vi "auto_sl.vi"() -> ()   [LabVIEW 2012, in "Mecanum Drive.lvrbt"]
uses:
  Mecanum Drive.lvrbt
  SubVIs/State_Typ.ctl
  <vilib>/NXT/HiTechnic/HiTechnic Controls/HiTechnic Port.ctl
  <vilib>/NXT/Block Support/NXT_InputPort.ctl
  SubVIs/auto_drive_TYP.ctl
  <vilib>/NXT/Hardware/Plugins/Tetrix DC Motor/TetrixDCMotorAddress.ctl
  <vilib>/NXT/Dual Mode Library/Display/drawNumber.vi
  <vilib>/NXT/NXTIO Xnodes/NXTIONodeSubVIs/TETRIX IO Check Battery.vi
  <vilib>/NXT/Dual Mode Library/Waits/Wait_Num(msec).vi
  <vilib>/NXT/NXTIO Xnodes/NXTIONodeSubVIs/TETRIX IO Reset Encoders.vi
  <vilib>/NXT/NXTIO Xnodes/NXTIONodeSubVIs/TETRIX IO Motor Status.vi
  <vilib>/NXT/NXTIO Xnodes/NXTIONodeSubVIs/TETRIX IO Stop DC Motors.vi
  <vilib>/NXT/Dual Mode Library/Sound/Tone.vi
  <vilib>/NXT/Dual Mode Library/Waits/Wait_Num.vi
  <vilib>/NXT/Subs/LVHSConnector.ctl
  <vilib>/NXT/NXTIO Xnodes/AddressXNode/NXTIOAddress.xnode
  <vilib>/NXT/NXTIO Xnodes/NXTIOXNode/NXTIO.xnode
  <vilib>/NXT/LegoClasses/BrickReference/BrickReference.lvclass
panel:
  out "Enabled":bool
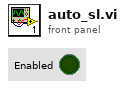
[diagram p1: front panel]
types:
  T1 = typedef "auto_drive_TYP.ctl" = cluster{"Left X":i8, "Left Y":i8, "Right X":i8, "Power (100)":i8, "Wait (ms)":u32, "Enc/Deg Target":i32, "Move Type":enum16{"Relative Degrees", "Wait", "Encoder"}}
  T2 = typedef "State_Typ.ctl" = enum16{"Stop", "Check for Position 3", "Check for Position 2", "Move", "Reset Enc", "Read Enc"}
  T3 = typedef "HiTechnic Port.ctl" = cluster{"Port":T4, "MUX Port":u8}
  T4 = typedef "NXT_InputPort.ctl" = u32
  T5 = typedef "TetrixDCMotorAddress.ctl" = i32
  T6 = typedef "LVHSConnector.ctl" = refnum<class "BrickReference.lvclass">
  T7 = cluster{"TetrixDCMotor":T5, "TetrixDCMotor 2":T5}
  T8 = cluster{"Direction (0-9)":i16, "Signal Strength (Array)":u8[]}
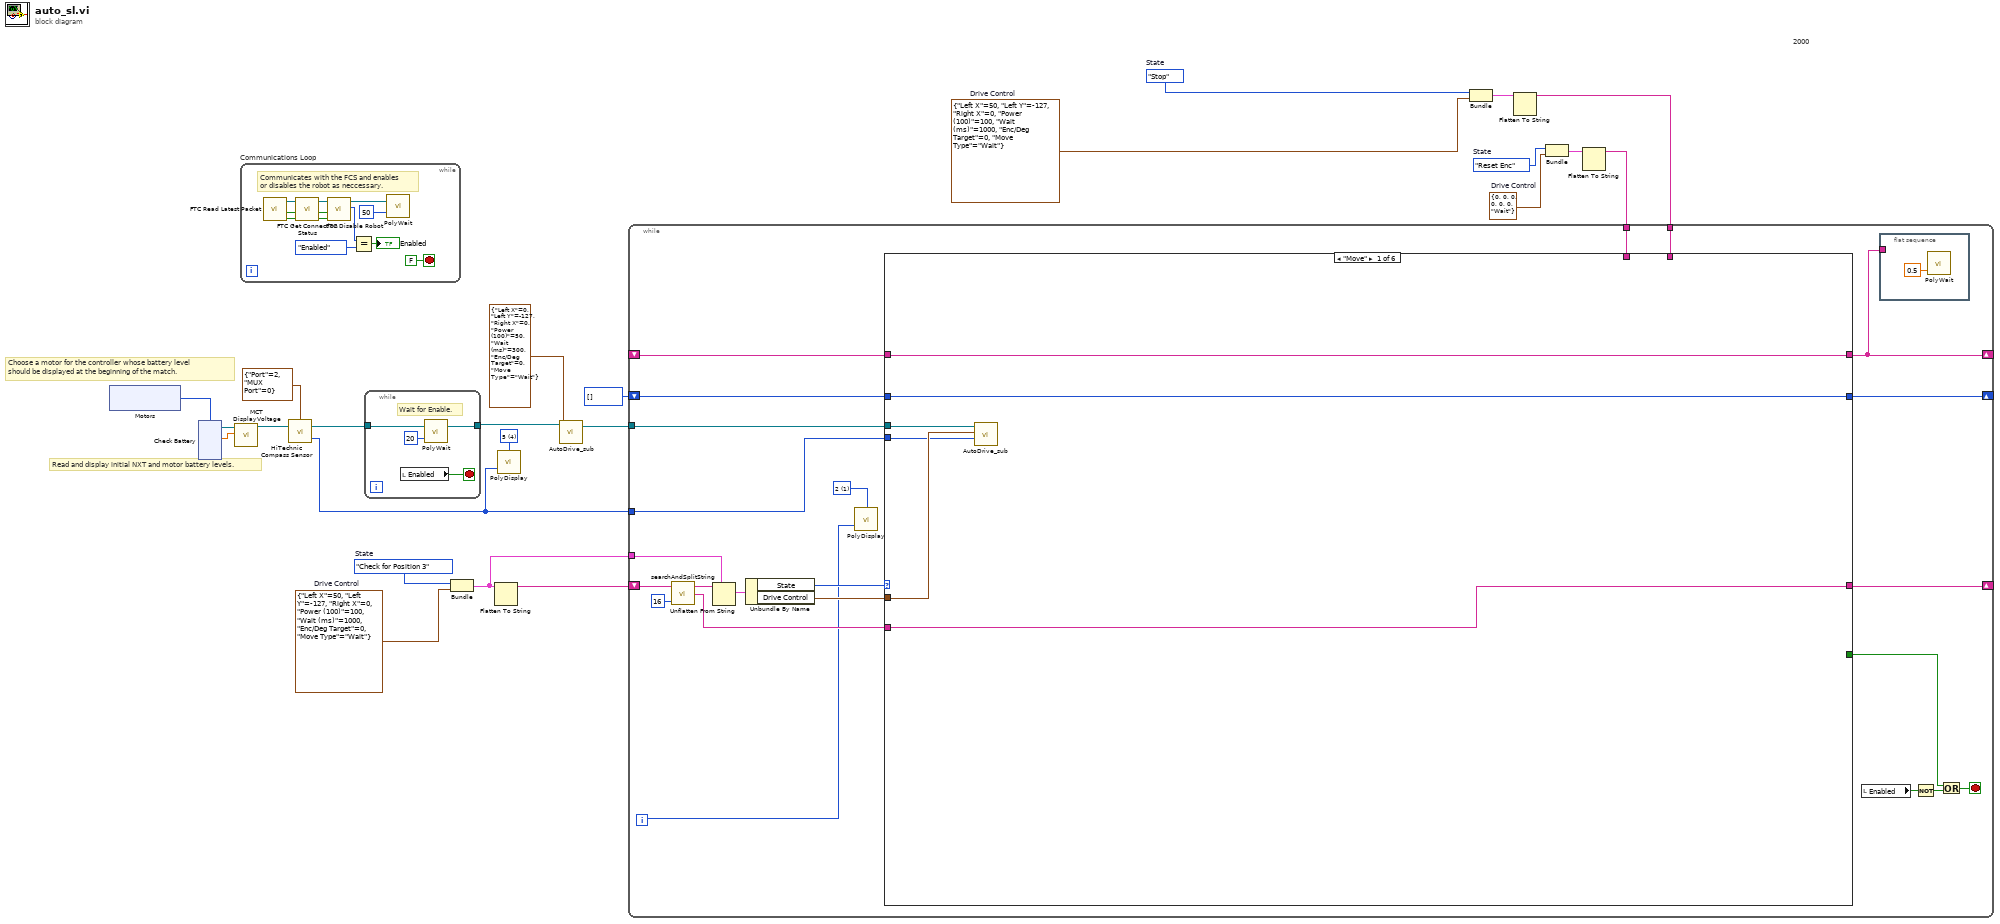
[diagram p0: block diagram]
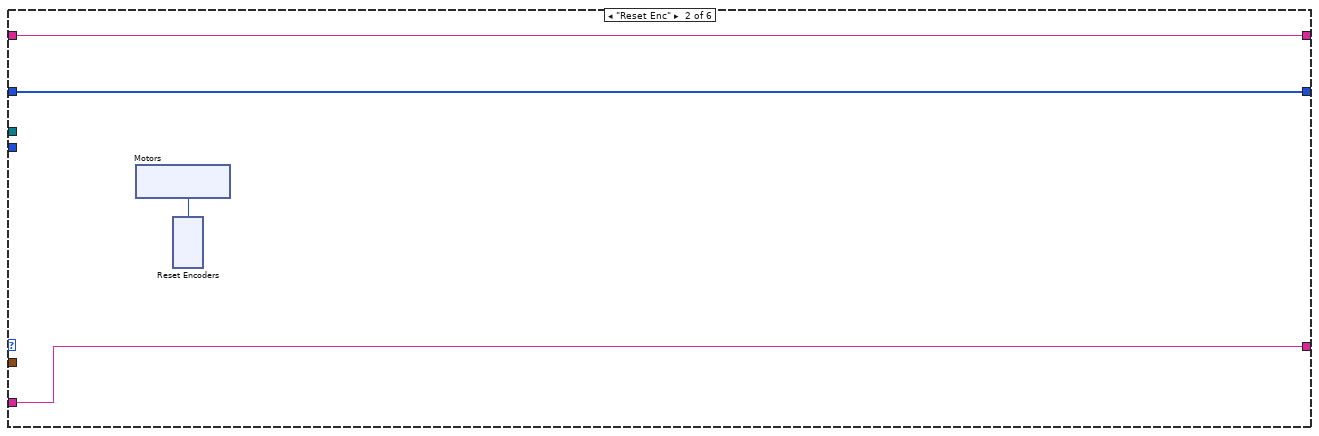
[diagram p2: hidden frame]
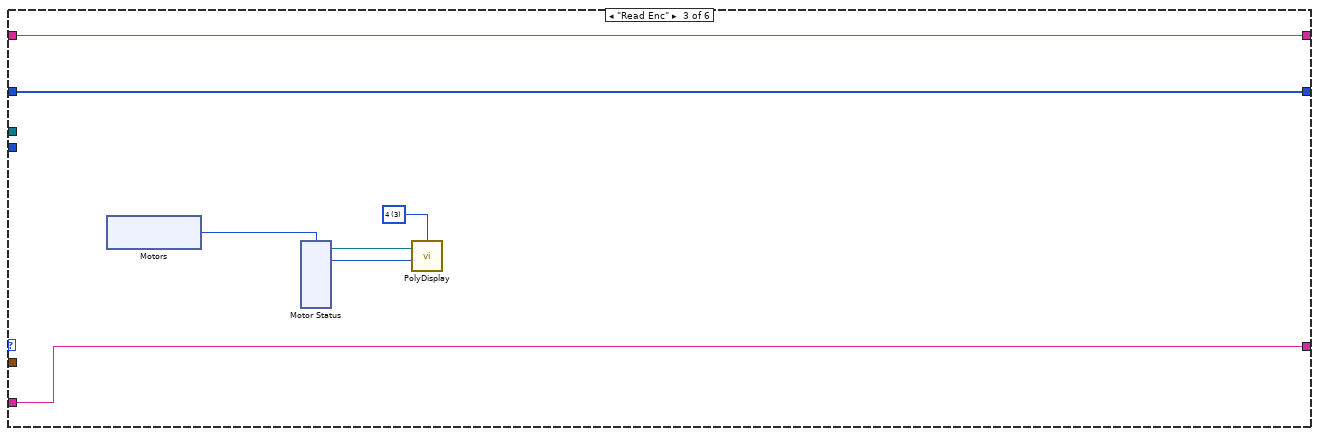
[diagram p3: hidden frame]
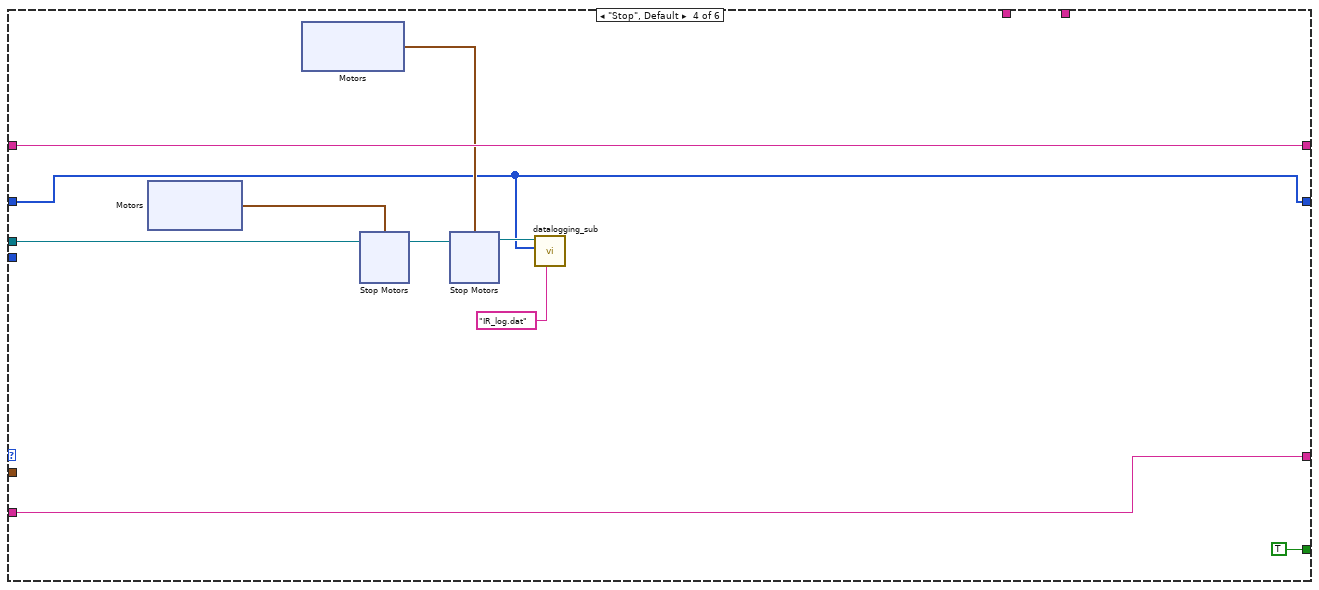
[diagram p4: hidden frame]
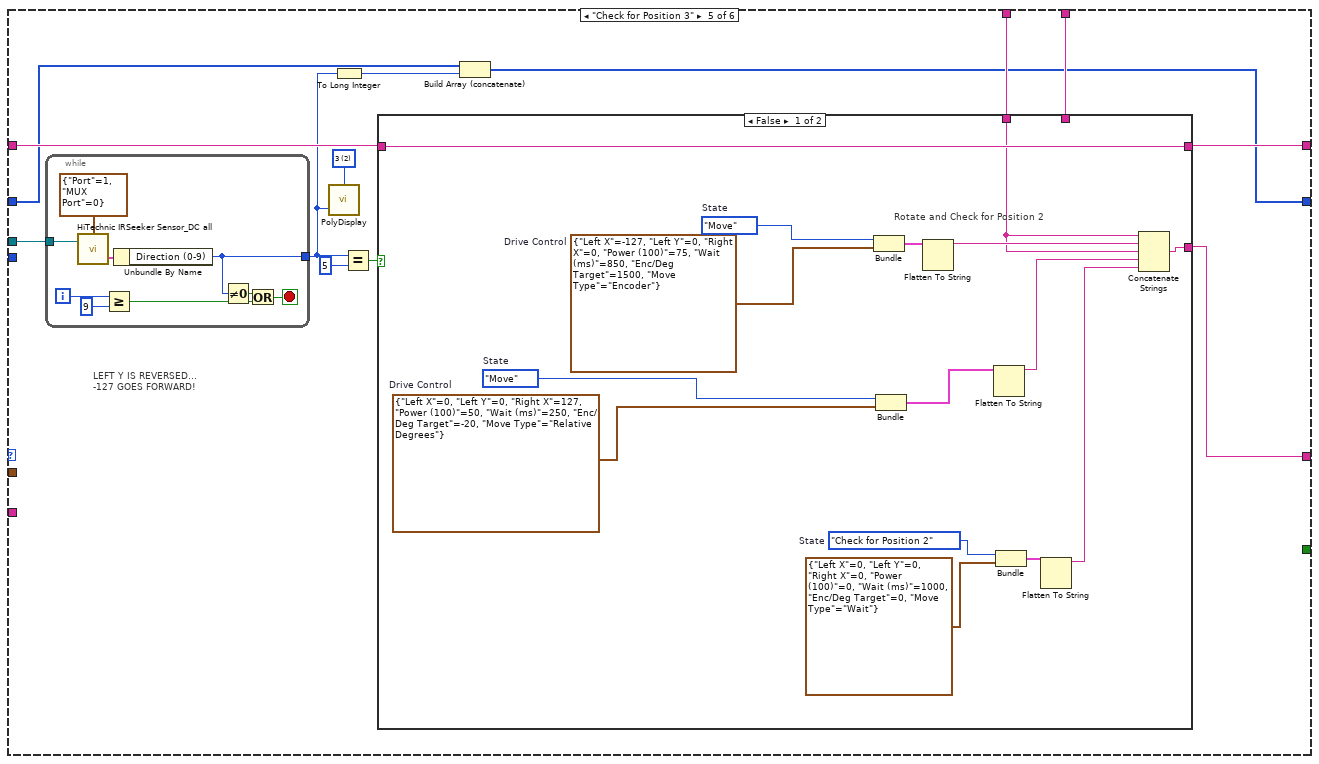
[diagram p5: hidden frame]
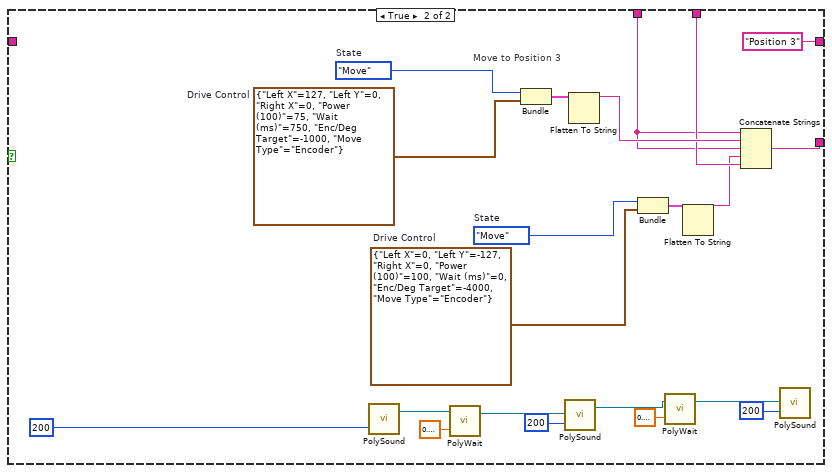
[diagram p6: hidden frame]
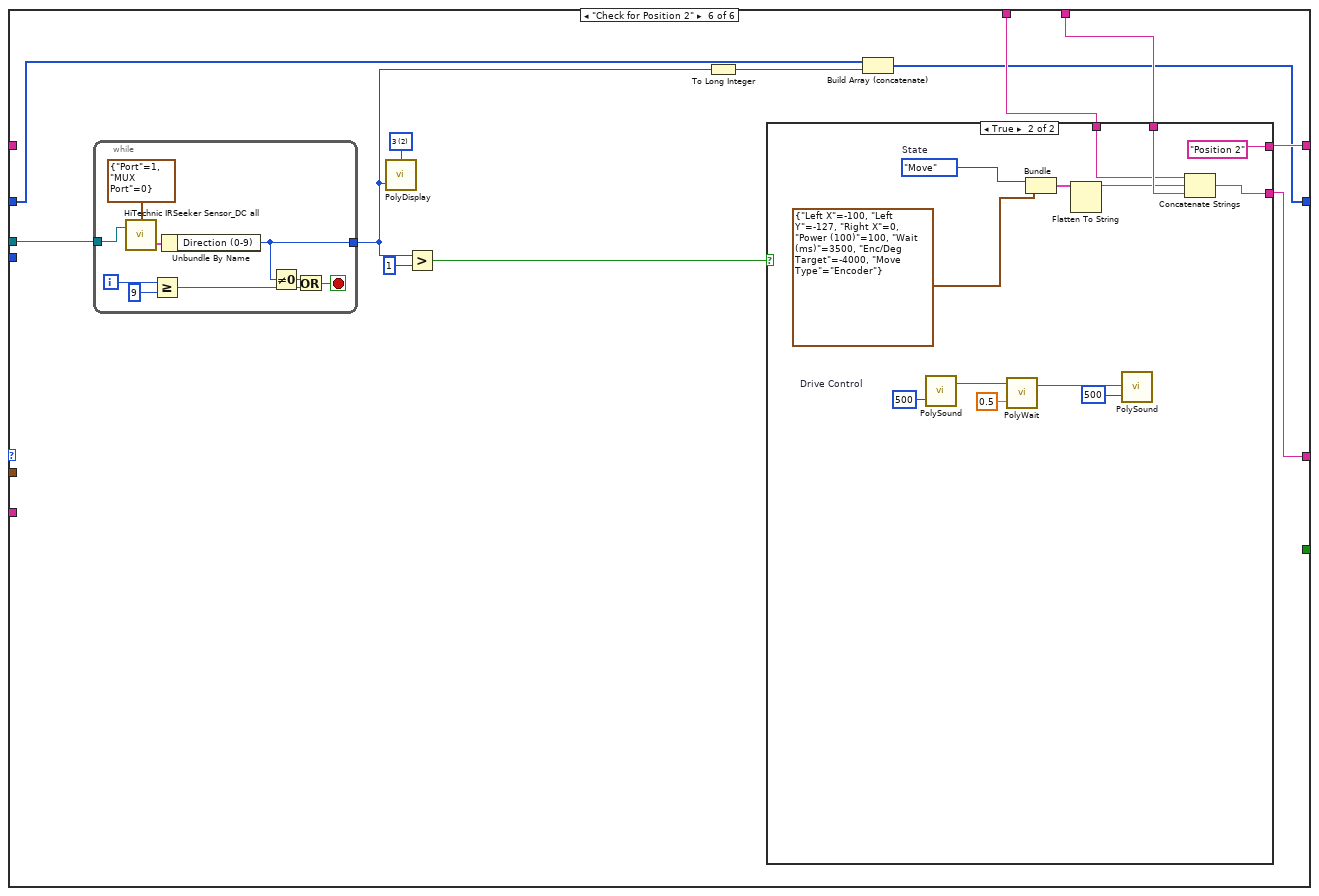
[diagram p7: hidden frame]
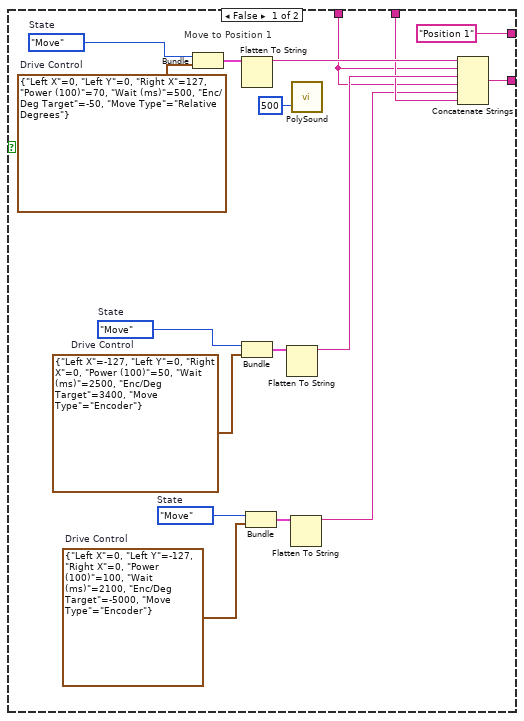
[diagram p8: hidden frame]
diagram:
  w1 = T1 {"Left X"=0, "Left Y"=0, "Right X"=0, "Power (100)"=0, "Wait (ms)"=0, "Enc/Deg Target"=0, "Move Type"=enum."Wait"}  # Drive Control
  w3 = State_Typ."Reset Enc"  # State
  w11 = T1 {"Left X"=50, "Left Y"=-127, "Right X"=0, "Power (100)"=100, "Wait (ms)"=1000, "Enc/Deg Target"=0, "Move Type"=enum."Wait"}  # Drive Control
  w12 = State_Typ."Stop"  # State
  w15 = i16 4 items=["1", "2", "3", "4", "5", "6", "7", "8", "9", "10", "11", "12"] ("Line")
  w24 = T1 {"Left X"=50, "Left Y"=-127, "Right X"=0, "Power (100)"=100, "Wait (ms)"=1000, "Enc/Deg Target"=0, "Move Type"=enum."Wait"}  # Drive Control
  w23 = State_Typ."Check for Position 3"  # State
  # "2000"
  # "Read and display initial NXT and motor battery levels."
  # "Choose a motor for the controller whose battery level \nshould be displayed at the beginning of the match."
  n1 = xnode "Motors"() -> ("Motor"=w20:T5)
  n2 = xnode "Check Battery"("Motors"=w20) -> ("Voltage 1"=w21:sgl, "NXT/EV3"=w22:T6)  [unwired: 1 in]
  n3 = call <vilib>:"MCT DisplayVoltage.vi"("Motor Voltage"=w21, "NXT"=w22) -> ("NXT"=w16:T6)  [unwired: 9 in]
  n4 = while "Communications Loop" {
    stop <- FALSE stop-if-true
    # "Communicates with the FCS and enables \nor disables the robot as neccessary."
    n5 = call <vilib>:"FTC Read Latest Packet.vi"() -> ("Packet Received?"=w34:bool, "Stopped?"=w33:bool, "NXT"=w36:T6)  [unwired: 6 in, 3 out]
    n6 = call <vilib>:"FTC Get Connection Status.vi"("Packet Received?"=w34, "Stopped?"=w33, "NXT"=w36) -> ("Online?"=w25:bool, "Stopped?"=w26:bool, "NXT"=w35:T6)  [unwired: 5 in]
    n7 = call <vilib>:"FTC Disable Robot.vi"("Online?"=w25, "Stopped?"=w26, "NXT"=w35) -> ("Enabled?"=w29:enum16{"Disabled", "Enabled"}, "NXT"=w31:T6)  [unwired: 3 in]
    n8 = Equal?(x=w29, y=enum16{"Disabled", "Enabled"}."Enabled") -> (x = y?=→"Enabled":bool)
    n9 = call-poly <vilib>:"PolyWait.vi"("Time (100 msec)"=u32 50 ("Time (msec)"), "NXT/EV3"=w31) -> ()  [unwired: 2 in, 1 out]
  }
  n10 = call <vilib>:"HiTechnic Compass Sensor.vi"("NXT/EV3"=w16, "Port/MUX"=T3 {"Port"=2, "MUX Port"=0}) -> ("Heading (degrees)"=w14:i16, "NXT/EV3"=w9:T6)  [unwired: 1 in]
  n11 = while {
    tunnel: [w38] -> w7
    tunnel: w9 -> [w37]
    stop <- w39 stop-if-true
    # "Wait for Enable."
    n12 = local read "Enabled"() -> (w39:bool)
    n13 = call-poly <vilib>:"PolyWait.vi"("Time (100 msec)"=u32 20 ("Time (msec)"), "NXT/EV3"=w37) -> ("NXT/EV3"=w38:T6)  [unwired: 2 in]
  }
  n14 = Bundle("State"=w23, "Drive Control"=w24) -> (w19:cluster{"State":T2, "Drive Control":T1})  [unwired: 1 in]
  n15 = Flatten To String(anything=w19) -> (data string=w18:string)  [unwired: 3 in, 2 out]
  n16 = call-poly <vilib>:"PolyDisplay.vi"("number"=w14, "Line"=w15) -> ()  [unwired: 2 in, 1 out]
  n17 = call "AutoDrive_sub.vi"("Drive Control"=T1 {"Left X"=0, "Left Y"=-127, "Right X"=0, "Power (100)"=50, "Wait (ms)"=300, "Enc/Deg Target"=0, "Move Type"=enum."Wait"}, "NXT/EV3"=w7) -> ("NXT/EV3 out"=w8:T6)  [unwired: 8 in, 1 out]
  n18 = Bundle("State"=w12, "Drive Control"=w11) -> (w13:cluster{"State":T2, "Drive Control":T1})  [unwired: 1 in]
  n19 = Flatten To String(anything=w13) -> (data string=w10:string)  [unwired: 3 in, 2 out]
  n20 = Bundle("State"=w3, "Drive Control"=w1) -> (w4:cluster{"State":T2, "Drive Control":T1})  [unwired: 1 in]
  n21 = Flatten To String(anything=w4) -> (data string=w2:string)  [unwired: 3 in, 2 out]
  n22 = while {
    tunnel: w8 -> [w63]
    shift-right: [w54] -> _
    shift-left: w18 -> [w52]
    tunnel: w19 -> [w55]
    shift-right: [w45] -> _
    shift-left: _ -> [w53]
    tunnel: w10 -> [w50]
    tunnel: w14 -> [w44]
    shift-right: [w43] -> _
    shift-left: i32[] [] -> [w42]
    tunnel: w2 -> [w41]
    i -> [w46]
    stop <- w62 stop-if-true
    w47 = i16 1 items=["1", "2", "3", "4", "5", "6", "7", "8", "9", "10", "11", "12"] ("Line")
    n23 = call <vilib>:"searchAndSplitString.vi"("offset (0)"=16 ("length (rest)"), "string"=w52) -> ("match + rest of string"=w51:string, "substring before match"=w57:string)  [unwired: 1 in, 1 out]
    n24 = Unflatten From String(type=w55, binary string=w57) -> (value=w56:cluster{"State":T2, "Drive Control":T1})  [unwired: 3 in, 2 out]
    n25 = Unbundle By Name(w56) -> ("State"=w48:T2, "Drive Control"=w58:T1)
    n26 = call-poly <vilib>:"PolyDisplay.vi"("number"=w46, "Line"=w47) -> ()  [unwired: 2 in, 1 out]
    n27 = case shown="\"Move\"" w48 {
      tunnel: w63 -> [w70 _ _ w105 w129 w180]
      tunnel: [_ _ _ TRUE _ _] -> w61
      tunnel: w58 -> [w69 _ _ _ _ _]
      tunnel: w51 -> [w68 w74 w86 w103 _ _]
      tunnel: [w68 w74 w86 w103 w125 w185] -> w54
      tunnel: [w67 w73 w85 w102 w128 w187] -> w45
      tunnel: w53 -> [w67 w73 w85 w102 w127 _]
      tunnel: w50 -> [_ _ _ _ w126 w186]
      tunnel: w44 -> [w66 _ _ _ _ _]
      tunnel: [w65 w71 w80 w97 w120 w183] -> w43
      tunnel: w42 -> [w65 w71 w80 w97 w121 w182]
      tunnel: w41 -> [_ _ _ _ w122 w184]
      frame "Move" {
        n28 = call "AutoDrive_sub.vi"("Target Heading (Degrees)"=w66, "Drive Control"=w69, "NXT/EV3"=w70) -> ()  [unwired: 7 in, 2 out]
      }
      frame "Reset Enc" {
        n29 = xnode "Motors"() -> ("Motor"=w72:T5)
        n30 = xnode "Reset Encoders"("Motors"=w72) -> ()  [unwired: 1 in, 1 out]
      }
      frame "Read Enc" {
        w82 = i16 3 items=["1", "2", "3", "4", "5", "6", "7", "8", "9", "10", "11", "12"] ("Line")
        n31 = xnode "Motors"() -> ("Motor"=w84:T5)
        n32 = xnode "Motor Status"("Motors"=w84) -> ("Position 1"=w83:i32, "NXT/EV3"=w81:T6)  [unwired: 1 in, 1 out]
        n33 = call-poly <vilib>:"PolyDisplay.vi"("number"=w83, "NXT/EV3"=w81, "Line"=w82) -> ()  [unwired: 1 in, 1 out]
      }
      frame "Stop", Default {
        n34 = xnode "Motors"() -> ("Motor"=w101:cluster{"TetrixDCMotor":T5, "TetrixDCMotor":T5})
        n35 = xnode "Motors"() -> ("Motor"=w100:cluster{"TetrixDCMotor":T5, "TetrixDCMotor":T5})
        n36 = xnode "Stop Motors"("Motors"=w101, "NXT/EV3"=w105) -> ("NXT/EV3"=w99:T6)
        n37 = xnode "Stop Motors"("Motors"=w100, "NXT/EV3"=w99) -> ("NXT/EV3"=w98:T6)
        n38 = call "datalogging_sub.vi"("Filename"="IR_log.dat", "Encoder Vals"=w97, "NXT/EV3 In"=w98) -> ()  [unwired: 8 in, 1 out]
      }
      frame "Check for Position 3" {
        w124 = i16 2 items=["1", "2", "3", "4", "5", "6", "7", "8", "9", "10", "11", "12"] ("Line")
        # "LEFT Y IS REVERSED...\n-127 GOES FORWARD!"
        n39 = while {
          tunnel: w129 -> [w138]
          tunnel: [w136] -> w119
          i -> [w134]
          stop <- w131 stop-if-true
          n40 = call <vilib>:"HiTechnic IRSeeker Sensor_DC all.vi"("NXT/EV3"=w138, "Port/MUX"=T3 {"Port"=1, "MUX Port"=0}) -> ("All Info"=w139:T8)  [unwired: 1 in, 1 out]
          n41 = Greater Or Equal?(x=w134, y=9 ("x")) -> (x >= y?=w132:bool)
          n42 = Unbundle By Name(w139) -> ("Direction (0-9)"=w136:i16)
          n43 = Not Equal To 0?(x=w136) -> (x != 0?=w135:bool)
          n44 = Or(x=w135, y=w132) -> (x .or. y?=w131:bool)
        }
        n45 = call-poly <vilib>:"PolyDisplay.vi"("number"=w119, "Line"=w124) -> ()  [unwired: 2 in, 1 out]
        n46 = To Long Integer(number=w119) -> (32bit integer=w118:i32)
        n47 = Equal?(x=w119, y=i16 5) -> (x = y?=w123:bool)
        n48 = case shown="False" w123 {
          tunnel: [w152 w168] -> w125
          tunnel: [w151 "Position 3"] -> w128
          tunnel: w127 -> [w151 _]
          tunnel: w126 -> [_ w166]
          tunnel: w122 -> [w144 w155]
          frame False {
            w141 = State_Typ."Check for Position 2"  # State
            w147 = T1 {"Left X"=0, "Left Y"=0, "Right X"=127, "Power (100)"=50, "Wait (ms)"=250, "Enc/Deg Target"=-20, "Move Type"=enum."Relative Degrees"}  # Drive Control
            w148 = State_Typ."Move"  # State
            w150 = T1 {"Left X"=-127, "Left Y"=0, "Right X"=0, "Power (100)"=75, "Wait (ms)"=850, "Enc/Deg Target"=1500, "Move Type"=enum."Encoder"}  # Drive Control
            w153 = State_Typ."Move"  # State
            # "Rotate and Check for Position 2"
            n49 = Bundle("State"=w153, "Drive Control"=w150) -> (w154:cluster{"State":T2, "Drive Control":T1})  [unwired: 1 in]
            n50 = Bundle("State"=w148, "Drive Control"=w147) -> (w149:cluster{"State":T2, "Drive Control":T1})  [unwired: 1 in]
            n51 = Flatten To String(anything=w154) -> (data string=w145:string)  [unwired: 3 in, 2 out]
            n52 = Flatten To String(anything=w149) -> (data string=w146:string)  [unwired: 3 in, 2 out]
            n53 = Bundle("State"=w141, "Drive Control"=T1 {"Left X"=0, "Left Y"=0, "Right X"=0, "Power (100)"=0, "Wait (ms)"=1000, "Enc/Deg Target"=0, "Move Type"=enum."Wait"}) -> (w143:cluster{"State":T2, "Drive Control":T1})  [unwired: 1 in]
            n54 = Flatten To String(anything=w143) -> (data string=w140:string)  [unwired: 3 in, 2 out]
            n55 = Concatenate Strings(w144, w145, w144, w146, w140) -> (w152:string)
          }
          frame True {
            w172 = T1 {"Left X"=0, "Left Y"=-127, "Right X"=0, "Power (100)"=100, "Wait (ms)"=0, "Enc/Deg Target"=-4000, "Move Type"=enum."Encoder"}  # Drive Control
            w173 = State_Typ."Move"  # State
            w175 = T1 {"Left X"=127, "Left Y"=0, "Right X"=0, "Power (100)"=75, "Wait (ms)"=750, "Enc/Deg Target"=-1000, "Move Type"=enum."Encoder"}  # Drive Control
            w174 = State_Typ."Move"  # State
            # "Move to Position 3"
            n56 = call-poly <vilib>:"PolySound.vi"("Duration (500 ms)"=u16 200) -> ("NXT/EV3"=w162:T6)  [unwired: 3 in]
            n57 = call-poly <vilib>:"PolyWait.vi"("Time (1 sec)"=sgl 0.2, "NXT/EV3"=w162) -> ("NXT/EV3"=w161:T6)  [unwired: 2 in]
            n58 = Bundle("State"=w174, "Drive Control"=w175) -> (w171:cluster{"State":T2, "Drive Control":T1})  [unwired: 1 in]
            n59 = call-poly <vilib>:"PolySound.vi"("Duration (500 ms)"=u16 200, "NXT/EV3"=w161) -> ("NXT/EV3"=w158:T6)  [unwired: 2 in]
            n60 = Flatten To String(anything=w171) -> (data string=w169:string)  [unwired: 3 in, 2 out]
            n61 = Bundle("State"=w173, "Drive Control"=w172) -> (w170:cluster{"State":T2, "Drive Control":T1})  [unwired: 1 in]
            n62 = call-poly <vilib>:"PolyWait.vi"("Time (1 sec)"=sgl 0.2, "NXT/EV3"=w158) -> ("NXT/EV3"=w157:T6)  [unwired: 2 in]
            n63 = Flatten To String(anything=w170) -> (data string=w156:string)  [unwired: 3 in, 2 out]
            n64 = Concatenate Strings(w155, w169, w155, w156, w166) -> (w168:string)
            n65 = call-poly <vilib>:"PolySound.vi"("Duration (500 ms)"=u16 200, "NXT/EV3"=w157) -> ()  [unwired: 2 in, 1 out]
          }
        }
        n66 = Build Array (concatenate)(w121, w118) -> (w120:i32[])
      }
      frame "Check for Position 2" {
        w178 = i16 2 items=["1", "2", "3", "4", "5", "6", "7", "8", "9", "10", "11", "12"] ("Line")
        n67 = while {
          tunnel: [w194] -> w176
          tunnel: w180 -> [w188]
          i -> [w192]
          stop <- w189 stop-if-true
          n68 = call <vilib>:"HiTechnic IRSeeker Sensor_DC all.vi"("NXT/EV3"=w188, "Port/MUX"=T3 {"Port"=1, "MUX Port"=0}) -> ("All Info"=w196:T8)  [unwired: 1 in, 1 out]
          n69 = Greater Or Equal?(x=w192, y=9 ("x")) -> (x >= y?=w190:bool)
          n70 = Unbundle By Name(w196) -> ("Direction (0-9)"=w194:i16)
          n71 = Not Equal To 0?(x=w194) -> (x != 0?=w193:bool)
          n72 = Or(x=w193, y=w190) -> (x .or. y?=w189:bool)
        }
        n73 = call-poly <vilib>:"PolyDisplay.vi"("number"=w176, "Line"=w178) -> ()  [unwired: 2 in, 1 out]
        n74 = Greater?(x=w176, y=i16 1) -> (0:w177:bool)
        n75 = To Long Integer(number=w176) -> (32bit integer=w181:i32)
        n76 = case shown="True" w177 {
          tunnel: [w210 w223] -> w185
          tunnel: ["Position 1" "Position 2"] -> w187
          tunnel: w186 -> [w202 w216]
          tunnel: w184 -> [w197 w214]
          frame False {
            w200 = T1 {"Left X"=0, "Left Y"=-127, "Right X"=0, "Power (100)"=100, "Wait (ms)"=2100, "Enc/Deg Target"=-5000, "Move Type"=enum."Encoder"}  # Drive Control
            w201 = State_Typ."Move"  # State
            w208 = T1 {"Left X"=-127, "Left Y"=0, "Right X"=0, "Power (100)"=50, "Wait (ms)"=2500, "Enc/Deg Target"=3400, "Move Type"=enum."Encoder"}  # Drive Control
            w209 = State_Typ."Move"  # State
            w212 = T1 {"Left X"=0, "Left Y"=0, "Right X"=127, "Power (100)"=70, "Wait (ms)"=500, "Enc/Deg Target"=-50, "Move Type"=enum."Relative Degrees"}  # Drive Control
            w213 = State_Typ."Move"  # State
            # "Move to Position 1"
            n77 = Bundle("State"=w213, "Drive Control"=w212) -> (w211:cluster{"State":T2, "Drive Control":T1})  [unwired: 1 in]
            n78 = Flatten To String(anything=w211) -> (data string=w204:string)  [unwired: 3 in, 2 out]
            n79 = Bundle("State"=w209, "Drive Control"=w208) -> (w207:cluster{"State":T2, "Drive Control":T1})  [unwired: 1 in]
            n80 = Bundle("State"=w201, "Drive Control"=w200) -> (w199:cluster{"State":T2, "Drive Control":T1})  [unwired: 1 in]
            n81 = Flatten To String(anything=w207) -> (data string=w206:string)  [unwired: 3 in, 2 out]
            n82 = Flatten To String(anything=w199) -> (data string=w198:string)  [unwired: 3 in, 2 out]
            n83 = call-poly <vilib>:"PolySound.vi"("Duration (500 ms)"=u16 500) -> ()  [unwired: 3 in, 1 out]
            n84 = Concatenate Strings(w204, w197, w206, w197, w198, w202) -> (w210:string)
          }
          frame True {
            w225 = T1 {"Left X"=-100, "Left Y"=-127, "Right X"=0, "Power (100)"=100, "Wait (ms)"=3500, "Enc/Deg Target"=-4000, "Move Type"=enum."Encoder"}  # Drive Control
            w224 = State_Typ."Move"  # State
            n85 = call-poly <vilib>:"PolySound.vi"("Duration (500 ms)"=u16 500) -> ("NXT/EV3"=w218:T6)  [unwired: 3 in]
            n86 = call-poly <vilib>:"PolyWait.vi"("Time (1 sec)"=sgl 0.5, "NXT/EV3"=w218) -> ("NXT/EV3"=w217:T6)  [unwired: 2 in]
            n87 = Bundle("State"=w224, "Drive Control"=w225) -> (w226:cluster{"State":T2, "Drive Control":T1})  [unwired: 1 in]
            n88 = Flatten To String(anything=w226) -> (data string=w215:string)  [unwired: 3 in, 2 out]
            n89 = call-poly <vilib>:"PolySound.vi"("Duration (500 ms)"=u16 500, "NXT/EV3"=w217) -> ()  [unwired: 2 in, 1 out]
            n90 = Concatenate Strings(w214, w215, w216) -> (w223:string)
          }
        }
        n91 = Build Array (concatenate)(w182, w181) -> (w183:i32[])
      }
    }
    n92 = local read "Enabled"() -> (w60:bool)
    n93 = flat-sequence {
      tunnel: w45 -> [_]
      frame #0 {
        n94 = call-poly <vilib>:"PolyWait.vi"("Time (1 sec)"=sgl 0.5) -> ()  [unwired: 3 in, 1 out]
      }
    }
    n95 = Not(x=w60) -> (.not. x?=w49:bool)
    n96 = Or(x=w61, y=w49) -> (x .or. y?=w62:bool)
  }
